vi "IS Create Bucket.vi"(8 "error in (no error)":errorcluster, 9 "Bucket Name (Optional)":string="LabVIEW-Created Bucket", 10 "Bucket Key (Optional)":string, 11 "IS Session In":T2={"Access Key"="", "HTTP Client Handle"=refnum}) -> (0 "error IO":errorcluster, 2 "IS Bucket Session":T1, 3 "IS Session Out":T2)   [LabVIEW 2017]
uses:
  Custom Data Types/IS Session.ctl
  <vilib>/httpClient/ClientHandle.ctl
  Custom Data Types/IS Bucket Session.ctl
  <vilib>/httpClient/POSTBuffer.vi
  <vilib>/httpClient/LabVIEWHTTPClient.lvlib
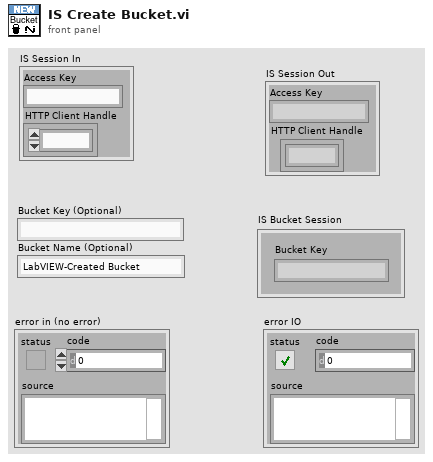
[diagram p1: front panel]
types:
  T1 = typedef "IS Bucket Session.ctl" = cluster{"Bucket Key":string}
  T2 = typedef "IS Session.ctl" = cluster{"Access Key":string, "HTTP Client Handle":T3}
  T3 = typedef "LabVIEWHTTPClient.lvlib/ClientHandle.ctl" = refnum<k1>
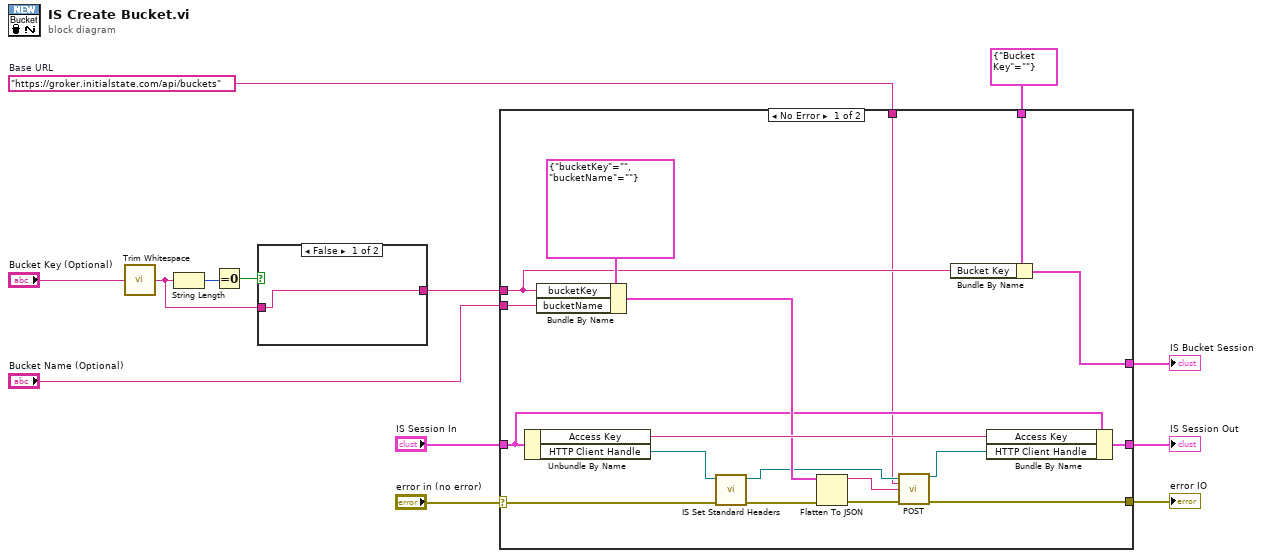
[diagram p0: block diagram]
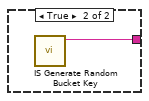
[diagram p2: hidden frame]
diagram:
  w2 = "https://groker.initialstate.com/api/buckets"  # Base URL
  n1 = call <vilib>:"Trim Whitespace.vi"("string"="Bucket Key (Optional)") -> ("trimmed string"=w6:string)  [unwired: 1 in]
  n2 = String Length(string=w6) -> (length=w9:i32)
  n3 = Equal To 0?(x=w9) -> (x = 0?=w8:bool)
  n4 = case shown="False" w8 {
    tunnel: [w14 w15] -> w5
    tunnel: w6 -> [w14 _]
    frame False {
    }
    frame True {
      n5 = call "IS Generate Random Bucket Key.vi"() -> ("string"=w15:string)  [unwired: 11 in]
    }
  }
  n6 = case shown="No Error" "error in (no error)" {
    selector: "error in (no error)" -> [w16 w36]
    tunnel: "IS Session In" -> [w19 w35]
    tunnel: [w33 w36] -> w10
    tunnel: [w30 w35] -> w11
    tunnel: w5 -> [w21 _]
    tunnel: "Bucket Name (Optional)" -> [w28 _]
    tunnel: [w22 w34] -> w4
    tunnel: T1 {"Bucket Key"=""} ("IS Bucket Session") -> [w20 w34]
    tunnel: w2 -> [w18 _]
    frame No Error {
      n7 = Unbundle By Name(w19) -> ("Access Key"=w32:string, "HTTP Client Handle"=w17:T3)
      n8 = Bundle By Name(cluster=cluster{"bucketKey":string, "bucketName":string} {"bucketKey"="", "bucketName"=""}, "bucketKey"=w21, "bucketName"=w28) -> (w27:cluster{"bucketKey":string, "bucketName":string})
      n9 = call "IS Set Standard Headers.vi"("error in (no error)"=w16, "client handle"=w17) -> ("error out"=w26:errorcluster, "client handle out"=w23:T3)  [unwired: 8 in]
      n10 = Flatten To JSON(anything=w27, error in (no error)=w26) -> (JSON string=w24:string, 11:w25:errorcluster)  [unwired: 1 in]
      n11 = call-poly <vilib>:"POST.vi"("client handle"=w23, "url"=w18, "buffer"=w24, "error in (no error)"=w25) -> ("client handle out"=w31:T3, "error out"=w33:errorcluster)  [unwired: 8 in, 2 out]
      n12 = Bundle By Name(cluster=w20, "Bucket Key"=w21) -> (w22:T1)
      n13 = Bundle By Name(cluster=w19, "Access Key"=w32, "HTTP Client Handle"=w31) -> (w30:T2)
    }
    frame Error {
    }
  }
  "IS Session Out" <- w11
  "error IO" <- w10
  "IS Bucket Session" <- w4
